vi "DecodeData.vi"(8 "Error In":errorcluster, 11 "Encoded Data":u8[](array[numeric])) -> (0 "Error Out":errorcluster, 2 "Check Syndrome":bool, 3 "Encoded Data Out":u8[](array[numeric]))   [LabVIEW 2010]
uses:
  RScode.dll
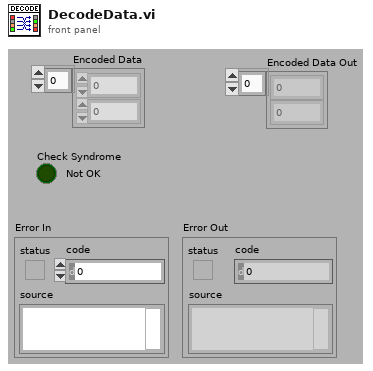
[diagram p1: front panel]
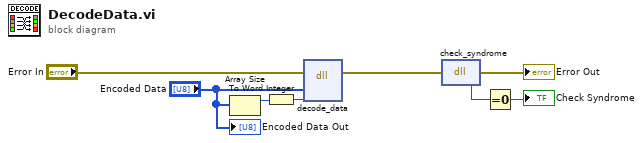
[diagram p0: block diagram]
diagram:
  n1 = Array Size(array="Encoded Data") -> (size(s)=w8:i32)
  n2 = To Word Integer(number=w8) -> (16bit integer=w7:i16)
  n3 = dll-call lib="Z:/Ted On My Mac/GitHub/Configurator/Source/Utilities/RScode/RScode.dll" fn="decode_data"(error in="Error In", "data"="Encoded Data", "bytes"=w7) -> (error out=w5:errorcluster)  [unwired: 5 in, 1 out]
  n4 = dll-call lib="Z:/Ted On My Mac/GitHub/Configurator/Source/Utilities/RScode/RScode.dll" fn="check_syndrome"(error in=w5) -> (error out=→"Error Out":errorcluster, "return type"=w3:i16)  [unwired: 2 in, 1 out]
  n5 = Equal To 0?(x=w3) -> (x = 0?=→"Check Syndrome":bool)
  "Encoded Data Out" <- "Encoded Data"
